vi "Kinect Gesture Processing.vi"() -> (0 "Kinect Enabled":bool, 1 "Skeleton Tracking State":T1[](array[typedef]), 2 "Joystick Data":T2)   [LabVIEW 2011]
doc: "This VI imlements the framework and scheduler for your robotics program. It should not be necessary to modify the framework. You are expected to add your code to the VIs called from Robot Main, the ones located in the Team Code within the project."
uses:
  <vilib>/addons/Kinect/SkeletonVertexTrackState.ctl
  <vilib>/addons/Kinect/Skeleton Vertex Index.ctl
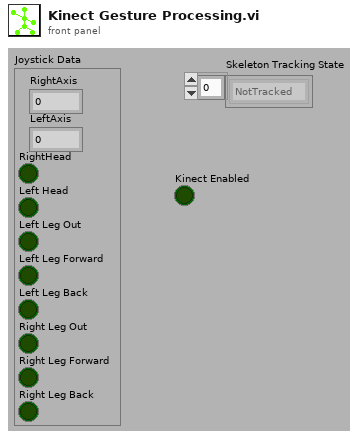
[diagram p1: front panel]
types:
  T1 = typedef "SkeletonVertexTrackState.ctl" = enum32{"NotTracked", "Inferred", "Tracked"}
  T2 = cluster{"RightAxis":dbl, "LeftAxis":dbl, "RightHead":bool, "Left Head":bool, "Left Leg Out":bool, "Left Leg Forward":bool, "Left Leg Back":bool, "Right Leg Out":bool, "Right Leg Forward":bool, "Right Leg Back":bool}
  T3 = typedef "Skeleton Vertex Index.ctl" = i32
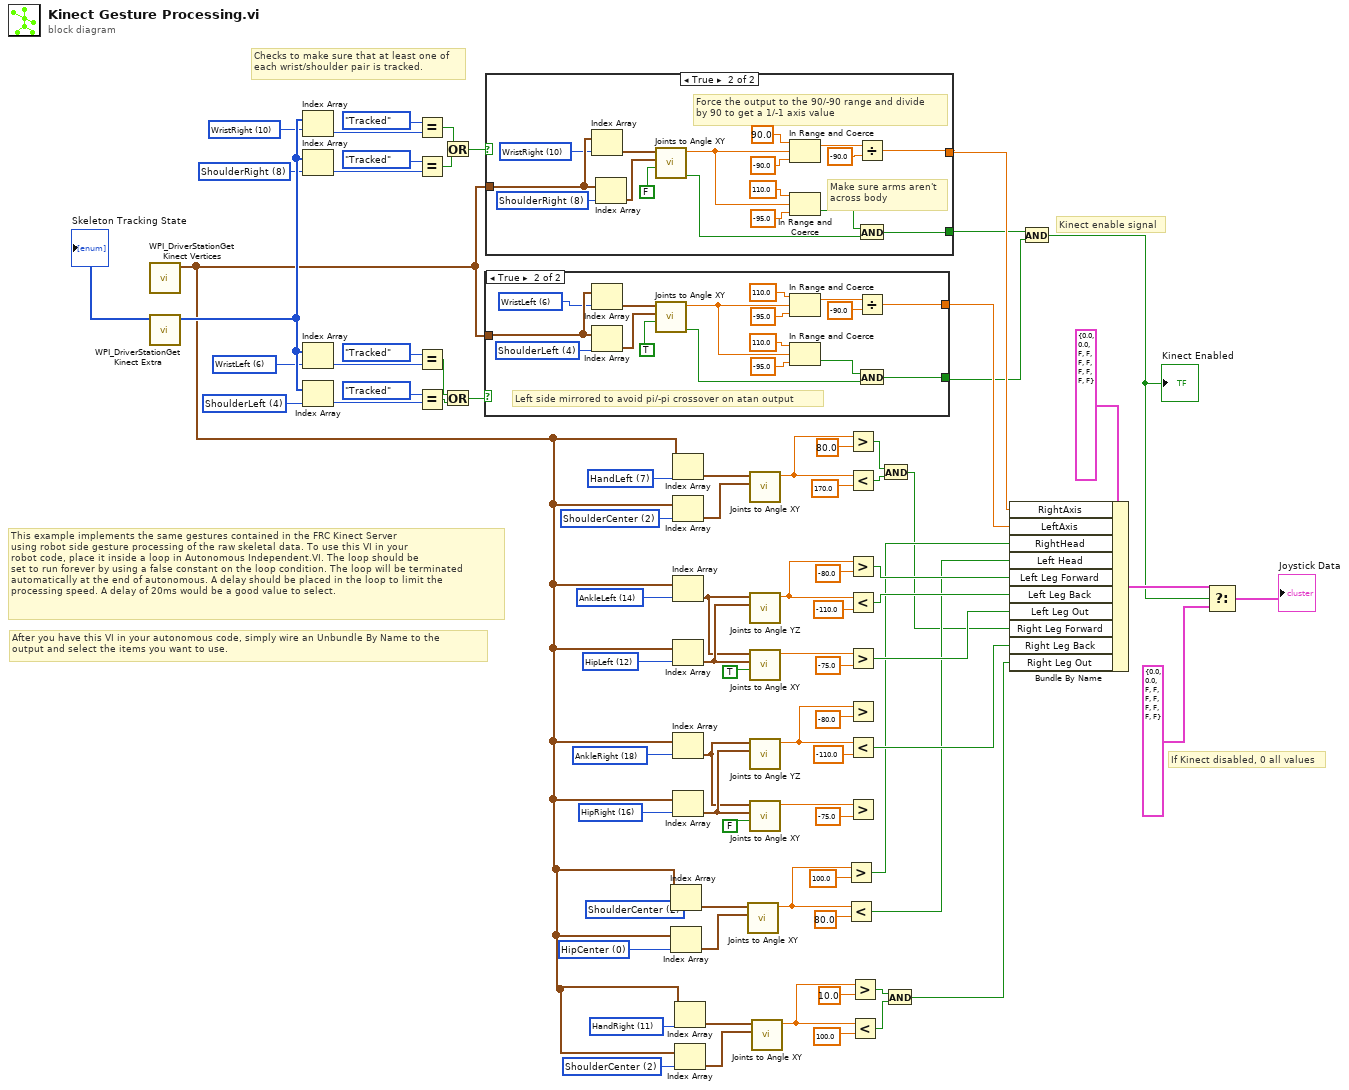
[diagram p0: block diagram]
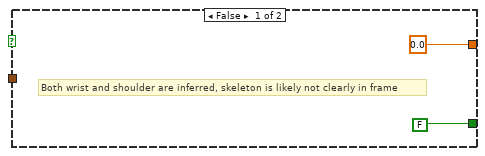
[diagram p2: hidden frame]
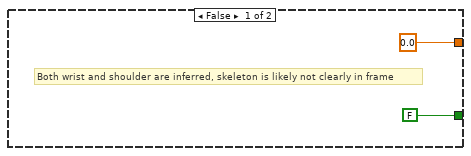
[diagram p3: hidden frame]
diagram:
  w5 = T3 2 items=["HipCenter", "Spine", "ShoulderCenter", "Head", "ShoulderLeft", "ElbowLeft", "WristLeft", "HandLeft", "ShoulderRight", "ElbowRight", "WristRight", "HandRight", "HipLeft", "KneeLeft", "AnkleLeft", "FootLeft", "HipRight", "KneeRight", "AnkleRight", "FootRight"] ("Skeleton Joints")
  w6 = T3 11 items=["HipCenter", "Spine", "ShoulderCenter", "Head", "ShoulderLeft", "ElbowLeft", "WristLeft", "HandLeft", "ShoulderRight", "ElbowRight", "WristRight", "HandRight", "HipLeft", "KneeLeft", "AnkleLeft", "FootLeft", "HipRight", "KneeRight", "AnkleRight", "FootRight"] ("Skeleton Joints")
  w17 = T3 0 items=["HipCenter", "Spine", "ShoulderCenter", "Head", "ShoulderLeft", "ElbowLeft", "WristLeft", "HandLeft", "ShoulderRight", "ElbowRight", "WristRight", "HandRight", "HipLeft", "KneeLeft", "AnkleLeft", "FootLeft", "HipRight", "KneeRight", "AnkleRight", "FootRight"] ("Skeleton Joints")
  w18 = T3 2 items=["HipCenter", "Spine", "ShoulderCenter", "Head", "ShoulderLeft", "ElbowLeft", "WristLeft", "HandLeft", "ShoulderRight", "ElbowRight", "WristRight", "HandRight", "HipLeft", "KneeLeft", "AnkleLeft", "FootLeft", "HipRight", "KneeRight", "AnkleRight", "FootRight"] ("Skeleton Joints")
  w26 = T3 16 items=["HipCenter", "Spine", "ShoulderCenter", "Head", "ShoulderLeft", "ElbowLeft", "WristLeft", "HandLeft", "ShoulderRight", "ElbowRight", "WristRight", "HandRight", "HipLeft", "KneeLeft", "AnkleLeft", "FootLeft", "HipRight", "KneeRight", "AnkleRight", "FootRight"] ("Skeleton Joints")
  w27 = T3 18 items=["HipCenter", "Spine", "ShoulderCenter", "Head", "ShoulderLeft", "ElbowLeft", "WristLeft", "HandLeft", "ShoulderRight", "ElbowRight", "WristRight", "HandRight", "HipLeft", "KneeLeft", "AnkleLeft", "FootLeft", "HipRight", "KneeRight", "AnkleRight", "FootRight"] ("Skeleton Joints")
  w25 = T3 12 items=["HipCenter", "Spine", "ShoulderCenter", "Head", "ShoulderLeft", "ElbowLeft", "WristLeft", "HandLeft", "ShoulderRight", "ElbowRight", "WristRight", "HandRight", "HipLeft", "KneeLeft", "AnkleLeft", "FootLeft", "HipRight", "KneeRight", "AnkleRight", "FootRight"] ("Skeleton Joints")
  w28 = T3 14 items=["HipCenter", "Spine", "ShoulderCenter", "Head", "ShoulderLeft", "ElbowLeft", "WristLeft", "HandLeft", "ShoulderRight", "ElbowRight", "WristRight", "HandRight", "HipLeft", "KneeLeft", "AnkleLeft", "FootLeft", "HipRight", "KneeRight", "AnkleRight", "FootRight"] ("Skeleton Joints")
  w29 = T3 2 items=["HipCenter", "Spine", "ShoulderCenter", "Head", "ShoulderLeft", "ElbowLeft", "WristLeft", "HandLeft", "ShoulderRight", "ElbowRight", "WristRight", "HandRight", "HipLeft", "KneeLeft", "AnkleLeft", "FootLeft", "HipRight", "KneeRight", "AnkleRight", "FootRight"] ("Skeleton Joints")
  w30 = T3 7 items=["HipCenter", "Spine", "ShoulderCenter", "Head", "ShoulderLeft", "ElbowLeft", "WristLeft", "HandLeft", "ShoulderRight", "ElbowRight", "WristRight", "HandRight", "HipLeft", "KneeLeft", "AnkleLeft", "FootLeft", "HipRight", "KneeRight", "AnkleRight", "FootRight"] ("Skeleton Joints")
  w31 = T3 4 items=["HipCenter", "Spine", "ShoulderCenter", "Head", "ShoulderLeft", "ElbowLeft", "WristLeft", "HandLeft", "ShoulderRight", "ElbowRight", "WristRight", "HandRight", "HipLeft", "KneeLeft", "AnkleLeft", "FootLeft", "HipRight", "KneeRight", "AnkleRight", "FootRight"] ("Skeleton Joints")
  w33 = T3 6 items=["HipCenter", "Spine", "ShoulderCenter", "Head", "ShoulderLeft", "ElbowLeft", "WristLeft", "HandLeft", "ShoulderRight", "ElbowRight", "WristRight", "HandRight", "HipLeft", "KneeLeft", "AnkleLeft", "FootLeft", "HipRight", "KneeRight", "AnkleRight", "FootRight"] ("Skeleton Joints")
  w32 = T3 8 items=["HipCenter", "Spine", "ShoulderCenter", "Head", "ShoulderLeft", "ElbowLeft", "WristLeft", "HandLeft", "ShoulderRight", "ElbowRight", "WristRight", "HandRight", "HipLeft", "KneeLeft", "AnkleLeft", "FootLeft", "HipRight", "KneeRight", "AnkleRight", "FootRight"] ("Skeleton Joints")
  w34 = T3 10 items=["HipCenter", "Spine", "ShoulderCenter", "Head", "ShoulderLeft", "ElbowLeft", "WristLeft", "HandLeft", "ShoulderRight", "ElbowRight", "WristRight", "HandRight", "HipLeft", "KneeLeft", "AnkleLeft", "FootLeft", "HipRight", "KneeRight", "AnkleRight", "FootRight"] ("Skeleton Joints")
  # "After you have this VI in your autonomous code, simply wire an Unbundle By Name to the\noutput and select the items you want to use."
  # "This example implements the same gestures contained in the FRC Kinect Server\nusing robot side gesture processing of the raw skeletal data. To use this VI in your\nrobot code, place it inside a loop in Autonomous Independent.VI. The loop should be\nset to run forever by using a false constant on the loop condition. The loop will be terminated\nautomatically at the end of autonomous. A delay should be placed in the loop to limit the \nprocessing speed. A delay of 20ms would be a good value to select."
  # "Checks to make sure that at least one of\neach wrist/shoulder pair is tracked."
  # "If Kinect disabled, 0 all values"
  # "Kinect enable signal"
  n1 = call <vilib>:"WPI_DriverStationGet Kinect Vertices.vi"() -> ("Skeleton Vertices"=w4:cluster{"x":sgl, "y":sgl, "z":sgl}[])  [unwired: 10 in, 1 out]
  n2 = call <vilib>:"WPI_DriverStationGet Kinect Extra.vi"() -> ("Skeleton Tracking State"=w50:T1[])  [unwired: 7 in, 4 out]
  "Skeleton Tracking State" <- w50
  n3 = Index Array(array=w50, index=w34) -> (element=w76:T1)
  n4 = Index Array(array=w50, index=w32) -> (element=w78:T1)
  n5 = Index Array(array=w50, index=w33) -> (element=w70:T1)
  n6 = Index Array(array=w50, index=w31) -> (element=w72:T1)
  n7 = Equal?(x=SkeletonVertexTrackState."Tracked", y=w76) -> (x = y?=w80:bool)
  n8 = Equal?(x=SkeletonVertexTrackState."Tracked", y=w78) -> (x = y?=w79:bool)
  n9 = Equal?(x=SkeletonVertexTrackState."Tracked", y=w70) -> (x = y?=w73:bool)
  n10 = Equal?(x=SkeletonVertexTrackState."Tracked", y=w72) -> (x = y?=w82:bool)
  n11 = Or(x=w80, y=w79) -> (x .or. y?=w81:bool)
  n12 = Or(x=w73, y=w82) -> (x .or. y?=w74:bool)
  n13 = case shown="True" w74 {
    tunnel: [0.0 w95] -> w54
    tunnel: w4 -> [_ w101]
    tunnel: [FALSE w91] -> w52
    frame False {
      # "Both wrist and shoulder are inferred, skeleton is likely not clearly in frame"
    }
    frame True {
      w85 = T3 4 items=["HipCenter", "Spine", "ShoulderCenter", "Head", "ShoulderLeft", "ElbowLeft", "WristLeft", "HandLeft", "ShoulderRight", "ElbowRight", "WristRight", "HandRight", "HipLeft", "KneeLeft", "AnkleLeft", "FootLeft", "HipRight", "KneeRight", "AnkleRight", "FootRight"] ("Skeleton Joints")
      w86 = T3 6 items=["HipCenter", "Spine", "ShoulderCenter", "Head", "ShoulderLeft", "ElbowLeft", "WristLeft", "HandLeft", "ShoulderRight", "ElbowRight", "WristRight", "HandRight", "HipLeft", "KneeLeft", "AnkleLeft", "FootLeft", "HipRight", "KneeRight", "AnkleRight", "FootRight"] ("Skeleton Joints")
      # "Left side mirrored to avoid pi/-pi crossover on atan output"
      n14 = Index Array(array=w101, index=w86) -> (element=w90:cluster{"x":sgl, "y":sgl, "z":sgl})
      n15 = Index Array(array=w101, index=w85) -> (element=w89:cluster{"x":sgl, "y":sgl, "z":sgl})
      n16 = call "Joints to Angle XY.vi"("Mirror"=TRUE, "Origin Joint"=w89, "Moving Joint"=w90) -> ("In-Plane"=w87:bool, "Angle"=w94:dbl)  [unwired: 7 in]
      n17 = In Range and Coerce(upper limit=110.0, x=w94, lower limit=-95.0) -> (coerced(x)=w100:dbl)  [unwired: 1 out]
      n18 = In Range and Coerce(upper limit=110.0, x=w94, lower limit=-95.0) -> (In Range?=w92:bool)  [unwired: 1 out]
      n19 = Divide(x=w100, y=-90.0) -> (x/y=w95:dbl)
      n20 = And(x=w92, y=w87) -> (x .and. y?=w91:bool)
    }
  }
  n21 = case shown="True" w81 {
    tunnel: [0.0 w116] -> w55
    tunnel: w4 -> [_ w120]
    tunnel: [FALSE w115] -> w53
    frame False {
      # "Both wrist and shoulder are inferred, skeleton is likely not clearly in frame"
    }
    frame True {
      w104 = T3 8 items=["HipCenter", "Spine", "ShoulderCenter", "Head", "ShoulderLeft", "ElbowLeft", "WristLeft", "HandLeft", "ShoulderRight", "ElbowRight", "WristRight", "HandRight", "HipLeft", "KneeLeft", "AnkleLeft", "FootLeft", "HipRight", "KneeRight", "AnkleRight", "FootRight"] ("Skeleton Joints")
      w105 = T3 10 items=["HipCenter", "Spine", "ShoulderCenter", "Head", "ShoulderLeft", "ElbowLeft", "WristLeft", "HandLeft", "ShoulderRight", "ElbowRight", "WristRight", "HandRight", "HipLeft", "KneeLeft", "AnkleLeft", "FootLeft", "HipRight", "KneeRight", "AnkleRight", "FootRight"] ("Skeleton Joints")
      # "Make sure arms aren't\nacross body"
      # "Force the output to the 90/-90 range and divide\nby 90 to get a 1/-1 axis value"
      n22 = Index Array(array=w120, index=w105) -> (element=w113:cluster{"x":sgl, "y":sgl, "z":sgl})
      n23 = Index Array(array=w120, index=w104) -> (element=w112:cluster{"x":sgl, "y":sgl, "z":sgl})
      n24 = call "Joints to Angle XY.vi"("Mirror"=FALSE, "Origin Joint"=w112, "Moving Joint"=w113) -> ("In-Plane"=w106:bool, "Angle"=w119:dbl)  [unwired: 7 in]
      n25 = In Range and Coerce(upper limit=90.0, x=w119, lower limit=-90.0) -> (coerced(x)=w117:dbl)  [unwired: 1 out]
      n26 = In Range and Coerce(upper limit=110.0, x=w119, lower limit=-95.0) -> (In Range?=w114:bool)  [unwired: 1 out]
      n27 = Divide(x=w117, y=-90.0) -> (x/y=w116:dbl)
      n28 = And(x=w114, y=w106) -> (x .and. y?=w115:bool)
    }
  }
  n29 = Index Array(array=w4, index=w18) -> (element=w20:cluster{"x":sgl, "y":sgl, "z":sgl})
  n30 = Index Array(array=w4, index=w17) -> (element=w19:cluster{"x":sgl, "y":sgl, "z":sgl})
  n31 = Index Array(array=w4, index=w30) -> (element=w49:cluster{"x":sgl, "y":sgl, "z":sgl})
  n32 = Index Array(array=w4, index=w29) -> (element=w48:cluster{"x":sgl, "y":sgl, "z":sgl})
  n33 = Index Array(array=w4, index=w28) -> (element=w44:cluster{"x":sgl, "y":sgl, "z":sgl})
  n34 = Index Array(array=w4, index=w25) -> (element=w45:cluster{"x":sgl, "y":sgl, "z":sgl})
  n35 = Index Array(array=w4, index=w27) -> (element=w46:cluster{"x":sgl, "y":sgl, "z":sgl})
  n36 = Index Array(array=w4, index=w26) -> (element=w47:cluster{"x":sgl, "y":sgl, "z":sgl})
  n37 = Index Array(array=w4, index=w6) -> (element=w8:cluster{"x":sgl, "y":sgl, "z":sgl})
  n38 = Index Array(array=w4, index=w5) -> (element=w7:cluster{"x":sgl, "y":sgl, "z":sgl})
  n39 = call "Joints to Angle XY.vi"("Origin Joint"=w19, "Moving Joint"=w20) -> ("Angle"=w22:dbl)  [unwired: 8 in, 1 out]
  n40 = call "Joints to Angle XY.vi"("Origin Joint"=w48, "Moving Joint"=w49) -> ("Angle"=w62:dbl)  [unwired: 8 in, 1 out]
  n41 = call "Joints to Angle YZ.vi"("Origin Joint"=w45, "Moving Joint"=w44) -> ("Angle"=w65:dbl)  [unwired: 9 in]
  n42 = call "Joints to Angle XY.vi"("Mirror"=TRUE, "Origin Joint"=w45, "Moving Joint"=w44) -> ("Angle"=w66:dbl)  [unwired: 7 in, 1 out]
  n43 = call "Joints to Angle YZ.vi"("Origin Joint"=w47, "Moving Joint"=w46) -> ("Angle"=w43:dbl)  [unwired: 9 in]
  n44 = call "Joints to Angle XY.vi"("Mirror"=FALSE, "Origin Joint"=w47, "Moving Joint"=w46) -> ("Angle"=w57:dbl)  [unwired: 7 in, 1 out]
  n45 = call "Joints to Angle XY.vi"("Origin Joint"=w7, "Moving Joint"=w8) -> ("Angle"=w10:dbl)  [unwired: 8 in, 1 out]
  n46 = Greater?(x=w22, y=100.0) -> (0:w16:bool)
  n47 = Less?(x=w22, y=80.0) -> (x < y?=w15:bool)
  n48 = Greater?(x=w62, y=80.0) -> (0:w13:bool)
  n49 = Less?(x=w62, y=170.0) -> (x < y?=w14:bool)
  n50 = Greater?(x=w65, y=-80.0) -> (0:w41:bool)
  n51 = Less?(x=w65, y=-110.0) -> (x < y?=w40:bool)
  n52 = Greater?(x=w66, y=-75.0) -> (0:w39:bool)
  n53 = Greater?(x=w43, y=-80.0) -> ()  [unwired: 1 out]
  n54 = Less?(x=w43, y=-110.0) -> (x < y?=w38:bool)
  n55 = Greater?(x=w57, y=-75.0) -> ()  [unwired: 1 out]
  n56 = Greater?(x=w10, y=10.0) -> (0:w3:bool)
  n57 = Less?(x=w10, y=100.0) -> (x < y?=w2:bool)
  n58 = And(x=w13, y=w14) -> (x .and. y?=w12:bool)
  n59 = And(x=w3, y=w2) -> (x .and. y?=w1:bool)
  n60 = Bundle By Name(cluster=T2 {"RightAxis"=0.0, "LeftAxis"=0.0, "RightHead"=FALSE, "Left Head"=FALSE, "Left Leg Out"=FALSE, "Left Leg Forward"=FALSE, "Left Leg Back"=FALSE, "Right Leg Out"=FALSE, "Right Leg Forward"=FALSE, "Right Leg Back"=FALSE} ("f"), "RightAxis"=w55, "LeftAxis"=w54, "RightHead"=w16, "Left Head"=w15, "Left Leg Forward"=w41, "Left Leg Back"=w40, "Left Leg Out"=w39, "Right Leg Forward"=w12, "Right Leg Back"=w38, "Right Leg Out"=w1) -> (w51:T2)
  n61 = And(x=w53, y=w52) -> (x .and. y?=w24:bool)
  "Kinect Enabled" <- w24
  n62 = Select(t=w51, s=w24, f=T2 {"RightAxis"=0.0, "LeftAxis"=0.0, "RightHead"=FALSE, "Left Head"=FALSE, "Left Leg Out"=FALSE, "Left Leg Forward"=FALSE, "Left Leg Back"=FALSE, "Right Leg Out"=FALSE, "Right Leg Forward"=FALSE, "Right Leg Back"=FALSE}) -> (s? t:f=→"Joystick Data":T2)
